vi "uClient_SetBroker.vi"(8 "error in (no error)":errorcluster, 10 "Broker":refnum<class "uTransport_uActor.lvclass">, 11 "uClient in":refnum<class "uClient.lvclass">) -> (0 "error out":errorcluster, 3 "uClient out":refnum<class "uClient.lvclass">)   [LabVIEW 2023, in "uLib.lvlib" / "uClient.lvclass"]
uses:
  uClient.lvclass
  uTransport/uTransport_uActor/uTransport_uActor.lvclass
  uClient.lvclass/uClient.ctl
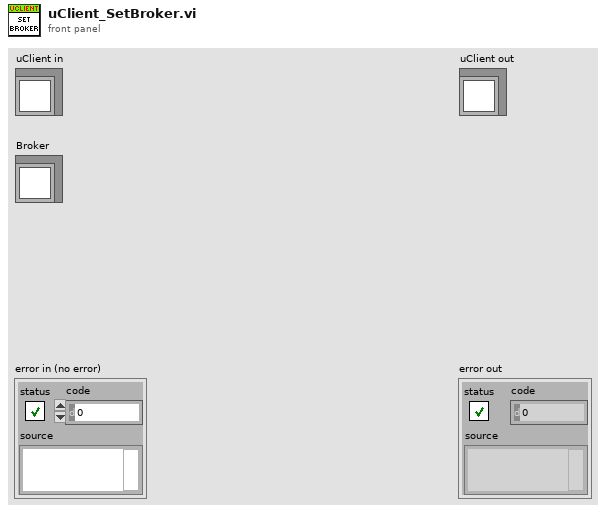
[diagram p1: front panel]
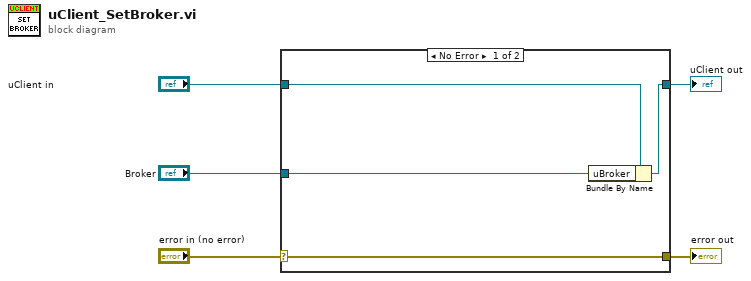
[diagram p0: block diagram]
diagram:
  n1 = case shown="No Error" "error in (no error)" {
    selector: "error in (no error)" -> [w9 w10]
    tunnel: [w9 w10] -> w4
    tunnel: [w7 w11] -> w2
    tunnel: "uClient in" -> [w8 w11]
    tunnel: "Broker" -> [w6 _]
    frame No Error {
      n2 = Bundle By Name(cluster=w8, "uBroker"=w6) -> (w7:refnum<class "uClient.lvclass">)
    }
    frame Error {
    }
  }
  "error out" <- w4
  "uClient out" <- w2
